vi "partial derivative with 2D encoded guassian.vi"(0 "Coefficients":dbl[](array[numeric]) format="%.2f", 2 "code":dbl format="%.2f", 3 "x":dbl format="%.2f", 4 "fit type":u16) -> (6 "Partial Derivative":dbl[](array[numeric]) format="%.5f")   [LabVIEW 2016]
doc: "This subprogram is derived from a subprogram contained in the National Instruments LabView advanced analysis library. The original subprogram is copyright National Instruments."
panel:
  # "Partial Derivative"
  # "This VI takes an input x along with a number of coefficients to use in the Target Func NonLin vi and does a numerical computation of the partial derivative of the function with repect to each coefficient at value x."
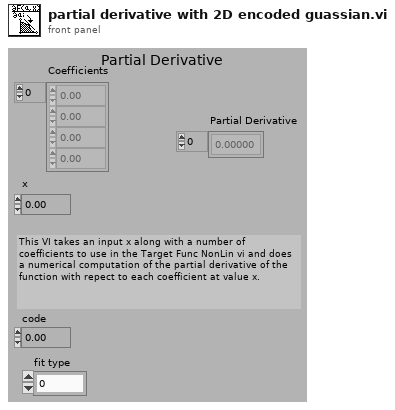
[diagram p1: front panel]
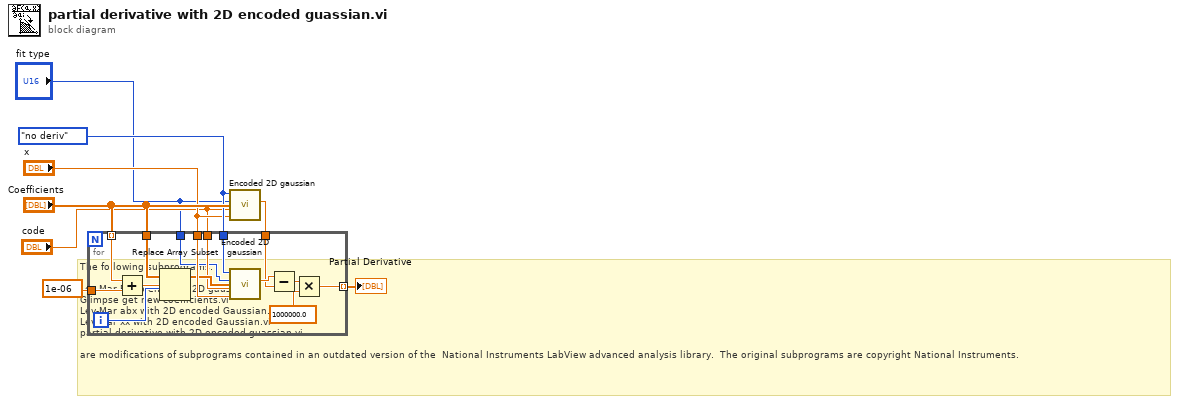
[diagram p0: block diagram]
diagram:
  w6 = enum16{"no deriv", "deriv"}."no deriv"
  # "The following subprograms:\n\nLev-Mar Fit to encoded 2D gaussian.vi\nGlimpse get new coefficients.vi\nLev-Mar abx with 2D encoded Gaussian.vi\nLev-Mar xx with 2D encoded Gaussian.vi\npartial derivative with 2D encoded guassian.vi\n\nare modifications of subprograms contained in an outdated version of the  National Instruments LabView advanced analysis library.  The original subprograms are copyright National Instruments."
  n1 = call "Encoded 2D gaussian.vi"("Coefficients"="Coefficients", "X"="x", "code"="code", "fit type"="fit type", "Flag"=w6) -> ("Y"=w4:dbl)  [unwired: 4 out]
  n2 = for {
    tunnel: "x" -> [w17]
    tunnel: [w21] -> w8 mode=indexing
    tunnel: "Coefficients" -> [w16] mode=indexing
    tunnel: "Coefficients" -> [w20]
    tunnel: w6 -> [w13]
    tunnel: w4 -> [w12]
    tunnel: 1e-06 -> [w11]
    tunnel: "code" -> [w10]
    tunnel: "fit type" -> [w9]
    i -> [w18]
    n3 = Add(x=w16, y=w11) -> (x+y=w19:dbl)
    n4 = Replace Array Subset(array=w20, new element=w19, index=w18) -> (w14:dbl[])
    n5 = call "Encoded 2D gaussian.vi"("Coefficients"=w14, "X"=w17, "code"=w10, "fit type"=w9, "Flag"=w13) -> ("Y"=w15:dbl)  [unwired: 4 out]
    n6 = Subtract(x=w15, y=w12) -> (x-y=w22:dbl)
    n7 = Multiply(x=w22, y=1000000.0) -> (x*y=w21:dbl)
  }
  "Partial Derivative" <- w8
